vi "Check VI condition.vi"(8 "error in (no error)":errorcluster, 11 "This VI":refnum<vi>) -> (0 "error out":errorcluster, 3 "Good To read BD?":bool)   [LabVIEW 2014, in "SmartPalette.lvlib"]
uses:
  SmartPalette.lvlib
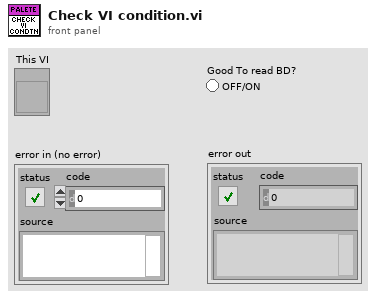
[diagram p1: front panel]
types:
  T1 = enum32{"Bad", "Idle", "Run top level", "Running"}
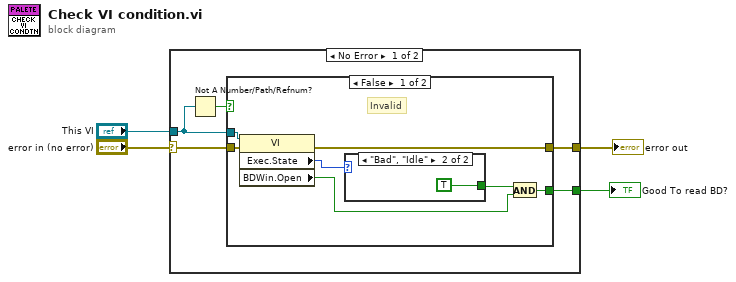
[diagram p0: block diagram]
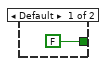
[diagram p2: hidden frame]
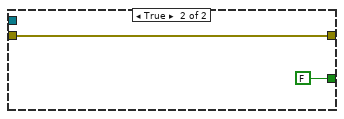
[diagram p3: hidden frame]
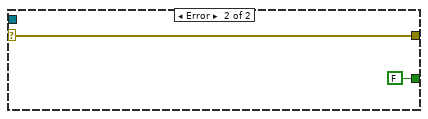
[diagram p4: hidden frame]
diagram:
  n1 = case shown="No Error" "error in (no error)" {
    selector: "error in (no error)" -> [w6 w22]
    tunnel: [w9 FALSE] -> w4
    tunnel: "This VI" -> [w8 _]
    tunnel: [w5 w22] -> w1
    frame No Error {
      n2 = Not A Number/Path/Refnum?(number/path/refnum=w8) -> (NaN/Path/Refnum?=w7:bool)
      n3 = case shown="False" w7 {
        tunnel: [w13 FALSE] -> w9
        tunnel: w8 -> [w12 _]
        tunnel: w6 -> [w11 w19]
        tunnel: [w10 w19] -> w5
        frame False {
          # "Invalid"
          n4 = property class="VI"(reference=w12, error in=w11) -> (error out=w10:errorcluster, "Exec.State"=w16:T1, "BDWin.Open"=w14:bool)  [unwired: 1 out]
          n5 = case shown="\"Bad\", \"Idle\"" w16 {
            tunnel: [FALSE TRUE] -> w15
            frame Default {
            }
            frame "Bad", "Idle" {
            }
          }
          n6 = And(x=w15, y=w14) -> (x .and. y?=w13:bool)
        }
        frame True {
        }
      }
    }
    frame Error {
    }
  }
  "Good To read BD?" <- w4
  "error out" <- w1
